vi "SEA-9811_ReceiverAndTransmitter_RT.vi"() -> ()   [LabVIEW 2017]
doc: "This example demonstrates the SEA 9811 ARINC-429 receiver and transmitter in normal mode. Transmitter and receiver can be used simultaneously. In order to receive transmitter data connect the transmitter line with the receiver lines at module's front connector. Please also refer to the FPGA VI.\n\n<B>Prerequisites:</B>\n1. NI CompactRIO\n2. SEA 9811\n3. In order to receive sent data: adapter that connects transmitter line with receiver line(s) (not included with the SEA 9811 module).\n\n<B>Instructions:</B>\n1. Run the VI.\n2. Enter data to be written in <B>Tx Data</B> and transmit it pressing the corresponding button.\n3. Observe that all 8 channels indicate that receiver FIFOs are NOT empty*.\n4. Observe that the sent data is shown in <B>Channel's Rx Data</B>*.\n5. Stop the VI.\n\n* only if an adequate adatper connects the transmitter lines with the receiver line(s).\n\nCopyright (c) 2013-2019 S.E.A. Datentechnik GmbH, Germany"
uses:
  <vilib>/rvi/interface/nirviReadWriteControl/nirviReadWriteControl.xnode
  <vilib>/rvi/interface/nirviCloseFPGA/nirviCloseFPGA.xnode
  <vilib>/rvi/interface/nirviMethod/nirviMethod.xnode
  SubVIs/SEA-9811_ReceiverAndTransmitter_RCR.ctl
  SubVIs/SEA-9811_ReceiverAndTransmitter_TCR.ctl
  <vilib>/rvi/errors/niLvFpgaAdjustHostInterfaceError.vi
  <vilib>/rvi/errors/niLvFpgaMergeErrorWithErrorCode.vi
  <vilib>/rvi/interface/nirviOpenFPGA/nirviOpenFPGA.xnode
  <vilib>/rvi/interface/Simulation/niFpgaSimulationCallBeginRW.vi
  <vilib>/FPGAPlugInAG/Dynamic/niLvFpga_ReadFifo_Dynamic.vi
  <vilib>/FPGAPlugInAG/Dynamic/niLvFpga_Reset_Dynamic.vi
  <vilib>/FPGAPlugInAG/Dynamic/niLvFpga_Run_Dynamic.vi
  <vilib>/rvi/interface/nirviMethod/StockFPGA_InlinedMethodWaitForSingleIRQ.vi
  <vilib>/FPGAPlugInAG/Dynamic/niLvFpga_WaitOnIrq_Dynamic.vi
  <vilib>/FPGAPlugInAG/Dynamic/niLvFpga_AcknowledgeIrq_Dynamic.vi
  Projekte/SEA/workspace_9811/cRIO_SEA_9811/Software/.SourceCode/Examples/SEA-9811_ReceiverAndTransmitter/SEA-9811_ReceiverAndTransmitter_FPGA.vi
  <vilib>/FPGAPlugInAG/Dynamic/niLvFpga_Close_Dynamic.vi
  SubVIs/SEA-9811_ReceiverAndTransmitter_RSR.ctl
  SubVIs/SEA-9811_ReceiverAndTransmitter_TSR.ctl
panel:
  in  "Rx Channel Number (0..7)":u8
  out "Transmitter Status Register (TSR)":T1={"TSR0: undefined"=FALSE, "TSR1: undefined"=FALSE, "TSR2: undefined"=FALSE, "TSR3: Transmitter FIFO empty?"=TRUE, "TSR4: Transmitter FIFO contains at least (TRUE)/less than (FALSE) 16 words"=FALSE, "TSR5: Transmitter FIFO full? (contains 32 words)"=FALSE, "TSR6: undefined"=FALSE, "TSR7: undefined"=FALSE}
  out "Receiver Status Register (RSR)":T2={"RSR0: FIFO channel 0 empty"=TRUE, "RSR1: FIFO channel 1 empty"=TRUE, "RSR2: FIFO channel 2 empty"=TRUE, "RSR3: FIFO channel 3 empty"=TRUE, "RSR4: FIFO channel 4 empty"=TRUE, "RSR5: FIFO channel 5 empty"=TRUE, "RSR6: FIFO channel 6 empty"=TRUE, "RSR7: FIFO channel 7 empty"=TRUE, "RSR8: FIFO channel 0 full"=FALSE, "RSR9: FIFO channel 1 full"=FALSE, "RSR10: FIFO channel 2 full"=FALSE, "RSR11: FIFO channel 3 full"=FALSE, "RSR12: FIFO channel 4 full"=FALSE, "RSR13: FIFO channel 5 full"=FALSE, "RSR14: FIFO channel 6 full"=FALSE, "RSR15: FIFO channel 7 full"=FALSE}
  in  "Rx Label Filter":T3
  in  "Transmit Cyclic":bool
  in  "Transmit Once":bool
  in  "Tx Data":u32 format="%08x"
  out "Channel's Rx Data":u32[](array[numeric]) format="%.0x"
  out "DMA Overflow":bool
  in  "stop":bool
  # "Please refer to VI description for instructions!"
  # "Receiver"
  # "Transmitter"
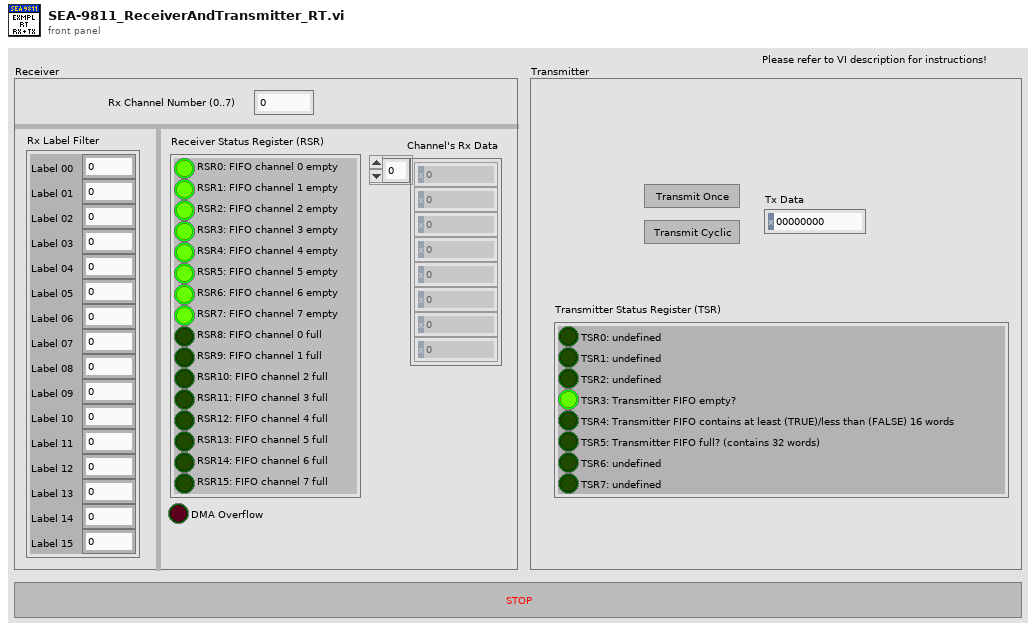
[diagram p1: front panel]
types:
  T1 = typedef "SEA-9811_ReceiverAndTransmitter_TSR.ctl" = cluster{"TSR0: undefined":bool, "TSR1: undefined":bool, "TSR2: undefined":bool, "TSR3: Transmitter FIFO empty?":bool, "TSR4: Transmitter FIFO contains at least (TRUE)/less than (FALSE) 16 words":bool, "TSR5: Transmitter FIFO full? (contains 32 words)":bool, "TSR6: undefined":bool, "TSR7: undefined":bool}
  T2 = typedef "SEA-9811_ReceiverAndTransmitter_RSR.ctl" = cluster{"RSR0: FIFO channel 0 empty":bool, "RSR1: FIFO channel 1 empty":bool, "RSR2: FIFO channel 2 empty":bool, "RSR3: FIFO channel 3 empty":bool, "RSR4: FIFO channel 4 empty":bool, "RSR5: FIFO channel 5 empty":bool, "RSR6: FIFO channel 6 empty":bool, "RSR7: FIFO channel 7 empty":bool, "RSR8: FIFO channel 0 full":bool, "RSR9: FIFO channel 1 full":bool, "RSR10: FIFO channel 2 full":bool, "RSR11: FIFO channel 3 full":bool, "RSR12: FIFO channel 4 full":bool, "RSR13: FIFO channel 5 full":bool, "RSR14: FIFO channel 6 full":bool, "RSR15: FIFO channel 7 full":bool}
  T3 = cluster{"Label 00":u8, "Label 01":u8, "Label 02":u8, "Label 03":u8, "Label 04":u8, "Label 05":u8, "Label 06":u8, "Label 07":u8, "Label 08":u8, "Label 09":u8, "Label 10":u8, "Label 11":u8, "Label 12":u8, "Label 13":u8, "Label 14":u8, "Label 15":u8}
  T4 = typedef "SEA-9811_ReceiverAndTransmitter_RCR.ctl" = cluster{"RCR0: Data rate = ARINC 429 High-Speed (0) or Low-Speed (1)":bool, "RCR1: not used":bool, "RCR2: Label recognition for this channel enabled (1) or disabled (0)":bool, "RCR3: Receiver channel disabled (1) or enabled (0)":bool, "RCR4: Odd parity check for this channel enabled (1) or disabled (0":bool, "RCR5: Receiver normal operation (1) or loopback mode (0)":bool, "RCR6: Receiver Decoder disabled (0) or enabled (1) -> ARINC bits 10 and 9 must match RCR7 and RCR8":bool, "RCR7: If receiver decoder is enabled (RCR6=1), the ARINC bit 10 must match this bit":bool, "RCR8: If receiver decoder is enabled (RCR6=1), the ARINC bit 9 must match this bit":bool, "RCR9: Label bit order for this channel non-reversed (1) or reversed (0)":bool, "RCR10: not used":bool, "RCR11: not used":bool, "RCR12: not used":bool, "RCR13: not used":bool, "RCR14: not used":bool, "RCR15: not used":bool}
  T5 = typedef "SEA-9811_ReceiverAndTransmitter_TCR.ctl" = cluster{"TCR0: not used":bool, "TCR1: not used":bool, "TCR2: not used":bool, "TCR3: Transmitter Parity Bit Enable: 32nd bit is parity (1) or data (0)":bool, "TCR4: not used":bool, "TCR5: not used":bool, "TCR6: not used":bool, "TCR7: not used":bool, "TCR8: not used":bool, "TCR9: Transmitter Parity Select: odd parity (0) or even parity (1)":bool, "TCR10: Transmitter Data Rate: ARINC 429 high-speed (0) or low-speed (1)":bool, "TCR11: ARINC Label Bit Order: label bit order reversed (0) or not reversed (1)":bool, "TCR12: Disable Line Driver: normal operation (0) or transmitter disabled (1)":bool, "TCR13: Tansmit whenever data is available in FIFO (1) or only start by instruction \"Enable Transmission\" (0)":bool, "TCR14: not used":bool, "TCR15: not used":bool}
  T6 = cluster{"Boolean array[0]":bool, "Boolean array[1]":bool, "Boolean array[2]":bool, "Boolean array[3]":bool, "Boolean array[4]":bool, "Boolean array[5]":bool, "Boolean array[6]":bool, "Boolean array[7]":bool, "Boolean array[8]":bool, "Boolean array[9]":bool, "Boolean array[10]":bool, "Boolean array[11]":bool, "Boolean array[12]":bool, "Boolean array[13]":bool, "Boolean array[14]":bool, "Boolean array[15]":bool}
  T7 = cluster{"Boolean array[0]":bool, "Boolean array[1]":bool, "Boolean array[2]":bool, "Boolean array[3]":bool, "Boolean array[4]":bool, "Boolean array[5]":bool, "Boolean array[6]":bool, "Boolean array[7]":bool}
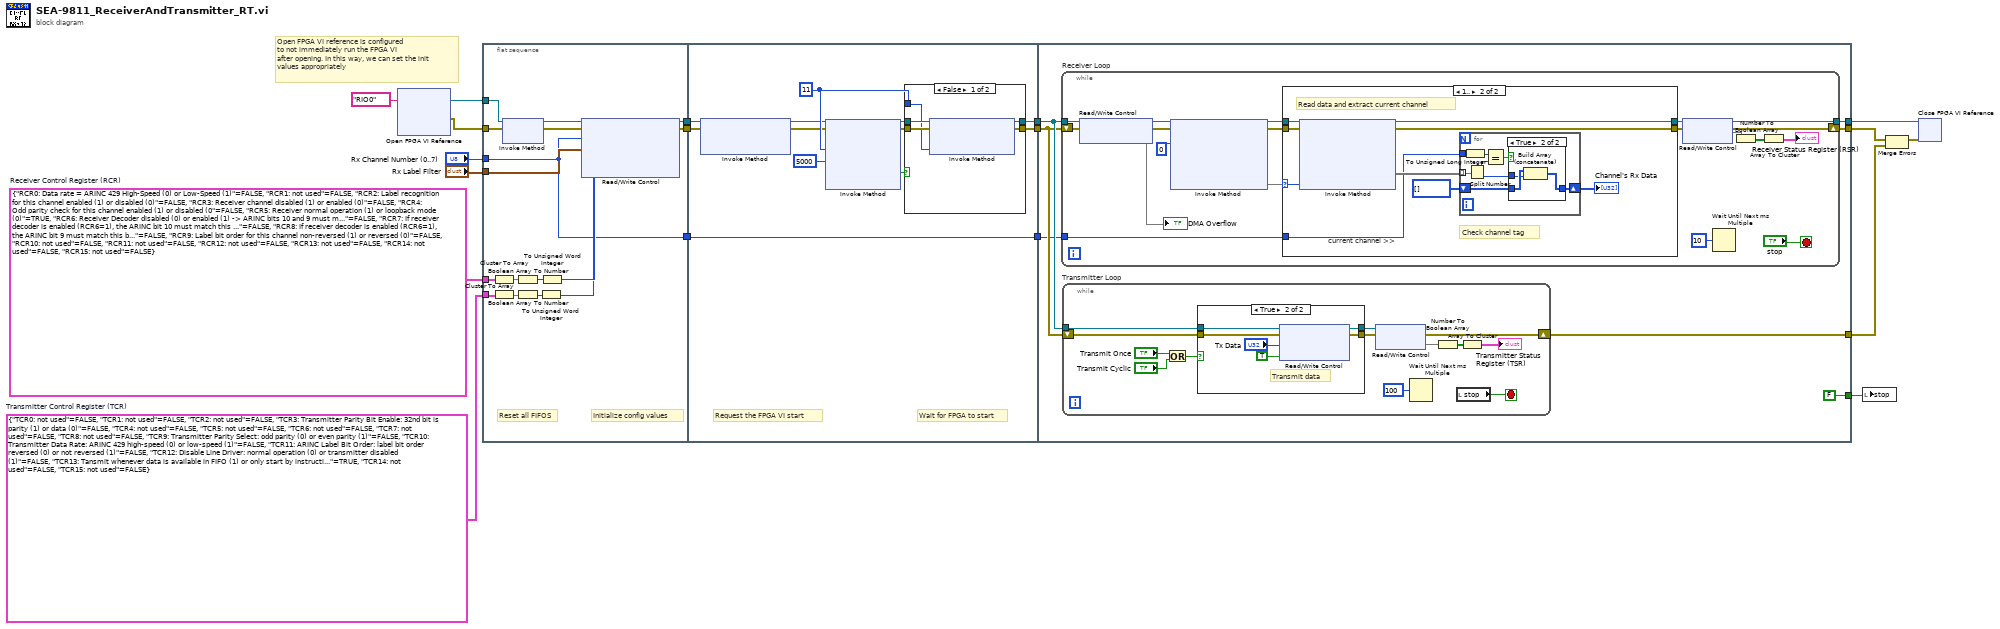
[diagram p0: block diagram]
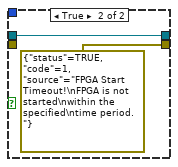
[diagram p2: hidden frame]
diagram:
  w14 = T4 {"RCR0: Data rate = ARINC 429 High-Speed (0) or Low-Speed (1)"=FALSE, "RCR1: not used"=FALSE, "RCR2: Label recognition for this channel enabled (1) or disabled (0)"=FALSE, "RCR3: Receiver channel disabled (1) or enabled (0)"=FALSE, "RCR4: Odd parity check for this channel enabled (1) or disabled (0"=FALSE, "RCR5: Receiver normal operation (1) or loopback mode (0)"=TRUE, "RCR6: Receiver Decoder disabled (0) or enabled (1) -> ARINC bits 10 and 9 must match RCR7 and RCR8"=FALSE, "RCR7: If receiver decoder is enabled (RCR6=1), the ARINC bit 10 must match this bit"=FALSE, "RCR8: If receiver decoder is enabled (RCR6=1), the ARINC bit 9 must match this bit"=FALSE, "RCR9: Label bit order for this channel non-reversed (1) or reversed (0)"=FALSE, "RCR10: not used"=FALSE, "RCR11: not used"=FALSE, "RCR12: not used"=FALSE, "RCR13: not used"=FALSE, "RCR14: not used"=FALSE, "RCR15: not used"=FALSE}  # Receiver Control Register (RCR)
  w13 = T5 {"TCR0: not used"=FALSE, "TCR1: not used"=FALSE, "TCR2: not used"=FALSE, "TCR3: Transmitter Parity Bit Enable: 32nd bit is parity (1) or data (0)"=FALSE, "TCR4: not used"=FALSE, "TCR5: not used"=FALSE, "TCR6: not used"=FALSE, "TCR7: not used"=FALSE, "TCR8: not used"=FALSE, "TCR9: Transmitter Parity Select: odd parity (0) or even parity (1)"=FALSE, "TCR10: Transmitter Data Rate: ARINC 429 high-speed (0) or low-speed (1)"=FALSE, "TCR11: ARINC Label Bit Order: label bit order reversed (0) or not reversed (1)"=FALSE, "TCR12: Disable Line Driver: normal operation (0) or transmitter disabled (1)"=FALSE, "TCR13: Tansmit whenever data is available in FIFO (1) or only start by instruction \"Enable Transmission\" (0)"=TRUE, "TCR14: not used"=FALSE, "TCR15: not used"=FALSE}  # Transmitter Control Register (TCR)
  # "Open FPGA VI reference is configured\nto not immediately run the FPGA VI\nafter opening. In this way, we can set the init\nvalues appropriately"
  n1 = xnode "Open FPGA VI Reference"("resource name"=tag "RIO0") -> ("FPGA VI Reference Out"=w2:refnum<k20>, "error out"=w1:errorcluster)  [unwired: 1 in]
  n2 = flat-sequence {
    tunnel: [w23] -> w9
    tunnel: [w24] -> w8
    tunnel: [w22] -> w6
    tunnel: "Rx Label Filter" -> [w26]
    tunnel: "Rx Channel Number (0..7)" -> [w22]
    tunnel: w14 -> [w34]
    tunnel: w13 -> [w29]
    tunnel: w2 -> [w20]
    tunnel: w1 -> [w19]
    tunnel: w9 -> [w45]
    tunnel: [w37] -> w11
    tunnel: w8 -> [w46]
    tunnel: [w36] -> w10
    tunnel: [w35] -> w7
    tunnel: w6 -> [w35]
    tunnel: [w60] -> w18
    tunnel: w11 -> [w58]
    tunnel: w10 -> [w59]
    tunnel: [w57] -> w12
    tunnel: [w56] -> w5
    tunnel: w7 -> [w55]
    tunnel: [FALSE ("stop")] -> w4
    frame #0 {
      # "Initialize config values"
      # "Reset all FIFOS"
      n3 = Cluster To Array(cluster=w34) -> (array=w33:bool[])
      n4 = Cluster To Array(cluster=w29) -> (array=w30:bool[])
      n5 = xnode "Invoke Method"("FPGA VI Reference In"=w20, "error in"=w19) -> ("FPGA VI Reference Out"=w21:refnum<k20>, "error out"=w25:errorcluster)
      n6 = Boolean Array To Number(Boolean array=w33) -> (number=w32:u32)
      n7 = Boolean Array To Number(Boolean array=w30) -> (number=w31:u32)
      n8 = To Unsigned Word Integer(number=w31) -> (unsigned 16bit integer=w27:u16)
      n9 = To Unsigned Word Integer(number=w32) -> (unsigned 16bit integer=w28:u16)
      n10 = xnode "Read/Write Control"("FPGA VI Reference In"=w21, "error in"=w25, "Rx Channel Number"=w22, "Rx Label Filter"=w26, "Rx Config Data (RCR)"=w28, "Tx Config Data (TCR)"=w27) -> ("FPGA VI Reference Out"=w24:refnum<k20>, "error out"=w23:errorcluster)
    }
    frame #1 {
      w42 = 11 ("IRQ Number (11)")
      # "Wait for FPGA to start"
      # "Request the FPGA VI start"
      n11 = xnode "Invoke Method"("FPGA VI Reference In"=w46, "error in"=w45) -> ("FPGA VI Reference Out"=w39:refnum<k20>, "error out"=w38:errorcluster)  [unwired: 1 in]
      n12 = xnode "Invoke Method"("FPGA VI Reference In"=w39, "error in"=w38, "IRQ Number(s)"=w42, "Timeout (ms)"=5000) -> ("FPGA VI Reference Out"=w44:refnum<k20>, "error out"=w43:errorcluster, "Timed Out"=w40:bool)  [unwired: 1 out]
      n13 = case shown="False" w40 {
        tunnel: w44 -> [w51 w53]
        tunnel: w43 -> [w50 _]
        tunnel: [w49 w53] -> w36
        tunnel: [w48 errorcluster {"status"=TRUE, "code"=1, "source"="FPGA Start Timeout!\nFPGA is not started\nwithin the specified\ntime period."} ("error in (no error)")] -> w37
        tunnel: w42 -> [w47 _]
        frame False {
          n14 = xnode "Invoke Method"("FPGA VI Reference In"=w51, "error in"=w50, "IRQ Number(s)"=w47) -> ("FPGA VI Reference Out"=w49:refnum<k20>, "error out"=w48:errorcluster)
        }
        frame True {
        }
      }
    }
    frame #2 {
      n15 = while "Receiver Loop" {
        tunnel: w59 -> [w85]
        tunnel: [w98] -> w60
        shift-right: [w97] -> w56
        shift-left: w58 -> [w84]
        tunnel: w55 -> [w82]
        stop <- "stop" stop-if-true
        n16 = xnode "Read/Write Control"("FPGA VI Reference In"=w85, "error in"=w84) -> ("FPGA VI Reference Out"=w87:refnum<k20>, "error out"=w86:errorcluster, "DMA Overflow"=→"DMA Overflow")
        n17 = xnode "Invoke Method"("FPGA VI Reference In"=w87, "error in"=w86, "Number of Elements"=u32 0) -> ("FPGA VI Reference Out"=w93:refnum<k20>, "error out"=w92:errorcluster, "Elements Remaining"=w83)  [unwired: 1 in, 1 out]
        n18 = case shown="1.." w83 {
          selector: w83 -> [_ w107]
          tunnel: w93 -> [w102 w111]
          tunnel: w92 -> [w101 w110]
          tunnel: [w102 w109] -> w90
          tunnel: [w101 w108] -> w89
          tunnel: w82 -> [_ w103]
          frame Default {
            # "not enough data to read"
          }
          frame 1.. {
            # "Check channel tag"
            # "Read data and extract current channel"
            # "current channel >>"
            n19 = xnode "Invoke Method"("FPGA VI Reference In"=w111, "error in"=w110, "Number of Elements"=w107) -> ("FPGA VI Reference Out"=w109:refnum<k20>, "error out"=w108:errorcluster, "Data"=w106:void[])  [unwired: 1 in, 1 out]
            n20 = for {
              tunnel: w106 -> [w119] mode=indexing
              shift-right: [w113] -> w104
              shift-left: u32[] [] -> [w114]
              tunnel: w103 -> [w117]
              n21 = To Unsigned Long Integer(number=w117) -> (unsigned 32bit integer=w112:u32)
              n22 = Split Number(x=w119) -> (hi(x)=w118:u16, lo(x)=w115:u16)
              n23 = Equal?(x=w112, y=w118) -> (x = y?=w116:bool)
              n24 = case shown="True" w116 {
                tunnel: w115 -> [_ w122]
                tunnel: w114 -> [w120 w123]
                tunnel: [w120 w121] -> w113
                frame False {
                }
                frame True {
                  n25 = Build Array (concatenate)(w123, w122) -> (w121:u32[])
                }
              }
            }
            "Channel's Rx Data" <- w104
          }
        }
        n26 = xnode "Read/Write Control"("FPGA VI Reference In"=w90, "error in"=w89) -> ("FPGA VI Reference Out"=w98:refnum<k20>, "error out"=w97:errorcluster, "Rx Status"=w96)
        n27 = Wait Until Next ms Multiple(millisecond multiple=u32 10) -> ()  [unwired: 1 out]
        n28 = Number To Boolean Array(number=w96) -> (Boolean array=w95:bool[])
        n29 = Array To Cluster(array=w95) -> (cluster=→"Receiver Status Register (RSR)":T6)
      }
      n30 = while "Transmitter Loop" {
        tunnel: w59 -> [w72]
        shift-right: [w64] -> w57
        shift-left: w58 -> [w71]
        stop <- w73 stop-if-true
        n31 = Or(x="Transmit Once", y="Transmit Cyclic") -> (x .or. y?=w70:bool)
        n32 = case shown="True" w70 {
          tunnel: w72 -> [w75 w81]
          tunnel: w71 -> [w74 w80]
          tunnel: [w75 w77] -> w66
          tunnel: [w74 w76] -> w65
          frame False {
          }
          frame True {
            # "Transmit data"
            n33 = xnode "Read/Write Control"("FPGA VI Reference In"=w81, "error in"=w80, "Tx Data"="Tx Data", "Transmit Data"=TRUE ("Trsanmit Data")) -> ("FPGA VI Reference Out"=w77:refnum<k20>, "error out"=w76:errorcluster)
          }
        }
        n34 = xnode "Read/Write Control"("FPGA VI Reference In"=w66, "error in"=w65) -> ("error out"=w64:errorcluster, "Tx Status"=w63)  [unwired: 1 out]
        n35 = Wait Until Next ms Multiple(millisecond multiple=u32 100) -> ()  [unwired: 1 out]
        n36 = Number To Boolean Array(number=w63) -> (Boolean array=w62:bool[])
        n37 = local read "stop"() -> (w73:bool)
        n38 = Array To Cluster(array=w62) -> (cluster=→"Transmitter Status Register (TSR)":T7)
      }
    }
  }
  n39 = local write "stop"(w4) -> ()
  n40 = Merge Errors(w5, w12) -> (w17:errorcluster)
  n41 = xnode "Close FPGA VI Reference"("FPGA VI Reference In"=w18, "error in"=w17) -> ()  [unwired: 1 out]
